vi "BASE.Create.vi"(8 "error in (no error)":errorcluster, 11 "Device.Simulation in":refnum<class "Device.Simulation.lvclass">) -> (0 "error out":errorcluster, 3 "Device.Simulation out":refnum<class "Device.Simulation.lvclass">)   [LabVIEW 2019, in "Device.Simulation.lvlib" / "Device.Simulation.lvclass"]
uses:
  Device.Simulation.lvclass
  Device.Simulation.lvclass/Device.Simulation.ctl
  Subsystems/BASE.Device/BASE.Device/BASE.Device.lvclass
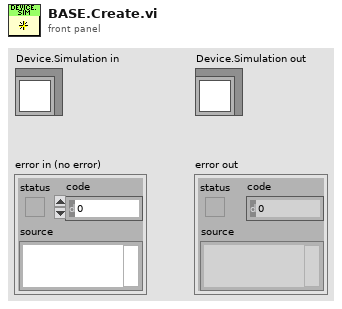
[diagram p1: front panel]
types:
  T1 = typedef "Device.Simulation.lvlib/Device.Simulation.lvclass/privateData--reference.ctl" = refnum<data-value>
  T2 = typedef "Device.Simulation.lvlib/Device.Simulation.lvclass/privateData--cluster.ctl" = cluster{"config":T3, "state":T4}
  T3 = typedef "Device.Simulation.lvlib/Device.Simulation.lvclass/config--cluster.ctl" = cluster{"Name":string, "Time to Connect (ms)":u32, "Time to Check Connection (ms)":u32, "Time to Disconnect (ms)":u32, "Time to Read State (ms)":u32}
  T4 = typedef "Device.Simulation.lvlib/Device.Simulation.lvclass/state--cluster.ctl" = cluster{"A1":dbl, "A2":dbl, "A3":dbl, "D1":bool, "D2":bool, "D3":bool}
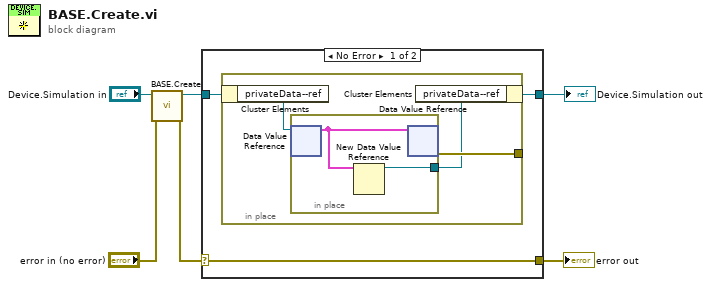
[diagram p0: block diagram]
diagram:
  n1 = call-parent "BASE.Create.vi"("error in (no error)"="error in (no error)", "BASE.Device in"="Device.Simulation in") -> ("error out"=w4:errorcluster, "BASE.Device out"=w2:refnum<class "Device.Simulation.lvclass">)  [unwired: 8 in]
  n2 = case shown="No Error" w4 {
    selector: w4 -> [w7 w15]
    tunnel: w2 -> [w9 w16]
    tunnel: [w8 w16] -> w1
    tunnel: [w7 w15] -> w3
    frame No Error {
      n3 = in-place {
        in-place-border: [w11] -> _
        n4 = in-place-cluster #1(w9) -> ("privateData--ref"=w12:T1)
        n5 = in-place {
          in-place-border: [w14] -> w10
          n6 = in-place-dvr #2(w12) -> (w13:T2)  [unwired: 1 out]
          n7 = New Data Value Reference(data value=w13) -> (data value reference=w14:refnum<data-value>)  [unwired: 1 in, 1 out]
          n8 = in-place-dvr #2(w13) -> (w11:errorcluster)  [unwired: 1 out]
        }
        n9 = in-place-cluster #1("privateData--ref"=w10) -> (w8:refnum<class "Device.Simulation.lvclass">)
      }
    }
    frame Error {
    }
  }
  "error out" <- w3
  "Device.Simulation out" <- w1
